vi "testTF.vi"() -> ()   [LabVIEW 2015]
uses:
  controls/ControlParams_TF.ctl
panel:
  in  "ControlParams":T1={"Umax "=0.0, "ymax"=0.0, "TsTicks"=0, "num"=[0.0, 0.0, 0.0, 0.0, 0.0, 0.0, 0.0, 0.0, 0.0], "den"=[0.0, 0.0, 0.0, 0.0, 0.0, 0.0, 0.0, 0.0, 0.0], "TF Order"=0, "num_ff"=[0.0, 0.0, 0.0, 0.0, 0.0, 0.0, 0.0, 0.0, 0.0], "den_ff"=[0.0, 0.0, 0.0, 0.0, 0.0, 0.0, 0.0, 0.0, 0.0], "TF_ff_order "=0, "ff_on"=FALSE}
  out "appended array":sgl[](array[numeric])
  in  "State In 2":sgl[](array[numeric])=[0.0, 0.0, 0.0, 0.0, 0.0, 0.0, 0.0, 0.0, 0.0]
  in  "r(k)":sgl[](array[numeric])
  out "u(k)":sgl[](array[numeric])
  # "Test the shift"
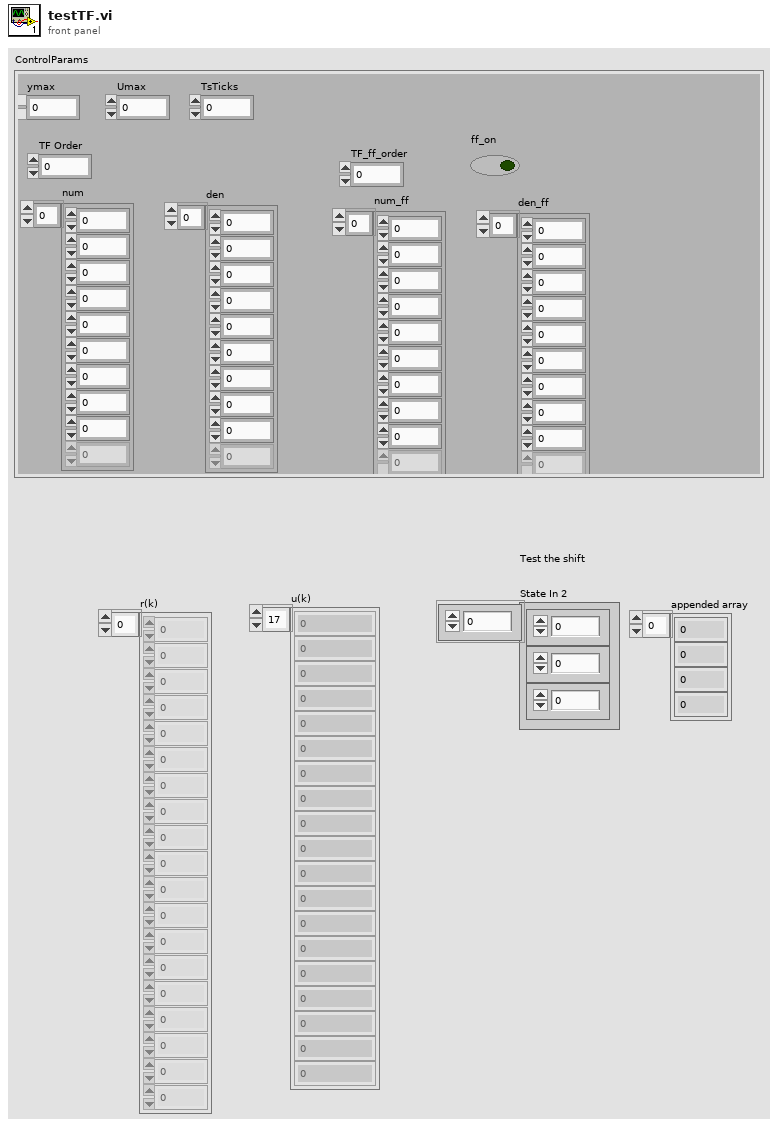
[diagram p1: front panel]
types:
  T1 = typedef "ControlParams_TF.ctl" = cluster{"Umax ":sgl, "ymax":sgl, "TsTicks":u32, "num":sgl[], "den":sgl[], "TF Order":u8, "num_ff":sgl[], "den_ff":sgl[], "TF_ff_order ":u8, "ff_on":bool}
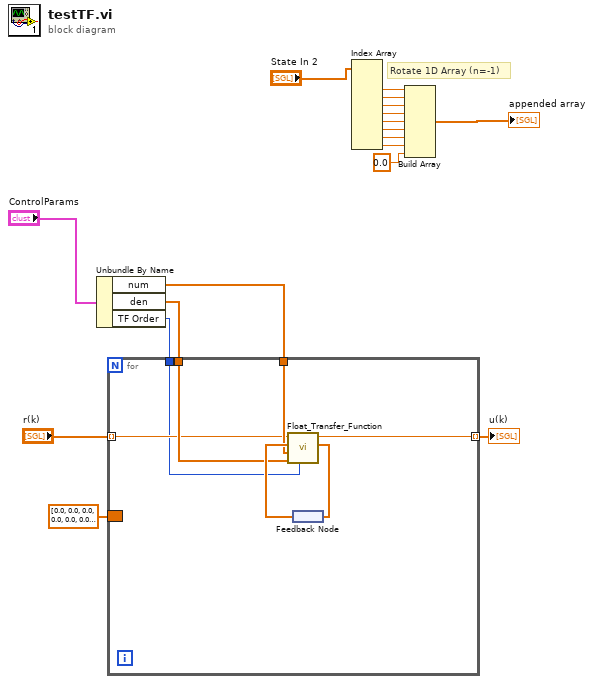
[diagram p0: block diagram]
diagram:
  # "Rotate 1D Array (n=-1)"
  n1 = Unbundle By Name("ControlParams") -> ("num"=w15:sgl[], "den"=w14:sgl[], "TF Order"=w13:u8)
  n2 = for {
    border: sgl[] [0.0, 0.0, 0.0, 0.0, 0.0, 0.0, 0.0, 0.0, 0.0] ("State Out") -> [_]
    tunnel: [w25] -> w17 mode=indexing
    tunnel: "r(k)" -> [w21] mode=indexing
    tunnel: w15 -> [w22]
    tunnel: w14 -> [w23]
    tunnel: w13 -> [w20]
    n3 = feedback #1() -> (w24:sgl[])
    n4 = call "Float_Transfer_Function.vi"("TF Order"=w20, "Den"=w23, "Num"=w22, "State In"=w24, "Input"=w21) -> ("State Out"=w19:sgl[], "Output"=w25:sgl)  [unwired: 4 in]
    n5 = feedback-in #1(w19) -> ()
  }
  "u(k)" <- w17
  n6 = Index Array(array="State In 2") -> (element #2=w12:sgl, element #3=w11:sgl, element #4=w10:sgl, element #5=w9:sgl, element #6=w8:sgl, element #7=w7:sgl, element #8=w6:sgl, element #9=w5:sgl)  [unwired: 9 in, 1 out]
  n7 = Build Array(w12, w11, w10, w9, w8, w7, w6, w5, sgl 0.0 ("element")) -> (→"appended array":sgl[])
